vi "Do.vi"(8 "error in (no error)":errorcluster, 10 "Series Enqueuer":refnum<class "Message Enqueuer.lvclass">, 11 "Sample PID Light in":refnum<class "Sample PID Light.lvclass">) -> (0 "error out":errorcluster, 3 "Sample PID Light out":refnum<class "Sample PID Light.lvclass">)   [LabVIEW 2023, in "Sample PID Light.lvclass"]
uses:
  Sample PID Light.lvclass
  D:/git/HAL/HAL GOOP4/Task/Task Base/Task Base.lvclass
  <vilib>/ActorFramework/Message Enqueuer/Message Enqueuer.lvclass
  Task/Task Base/Task Base.lvclass/Task Base.ctl
  Series/ISeries Actor/ISeries Actor Messages/Point Data Updated Msg/Point Data Updated Msg.lvclass/Point Data Updated Msg.ctl
  <vilib>/ActorFramework/Message Enqueuer/Message Enqueuer.lvclass/Message Enqueuer.ctl
  <vilib>/ActorFramework/Message Enqueuer/Enqueue.vi
  Series/ISeries Actor/ISeries Actor Messages/Point Data Updated Msg/Point Data Updated Msg.lvclass
  C:/Program Files/National Instruments/LabVIEW 2023/vi.lib/ActorFramework/Message/Message.lvclass
  <vilib>/addons/control/pid/pid.llb/PID (DBL).vi
  <vilib>/Utility/LVClass/Get LV Class Name.vi
  <resource>/AFDebug/Generate Trace for Message.vi
  <vilib>/ActorFramework/Message Priority Queue/Priority Enqueue.vi
  Task/Task Base/Task Base.lvclass
  <vilib>/addons/control/pid/NI_PID_pid.lvlib
  Measure and Stimulus Subsystems/Measure and Stimulus Subsystems.lvclass
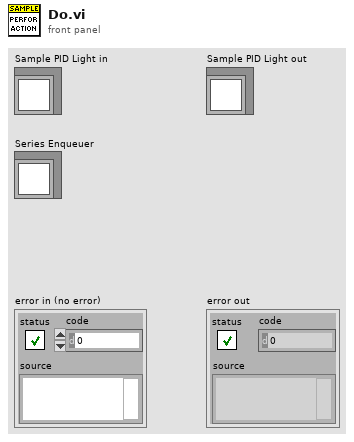
[diagram p1: front panel]
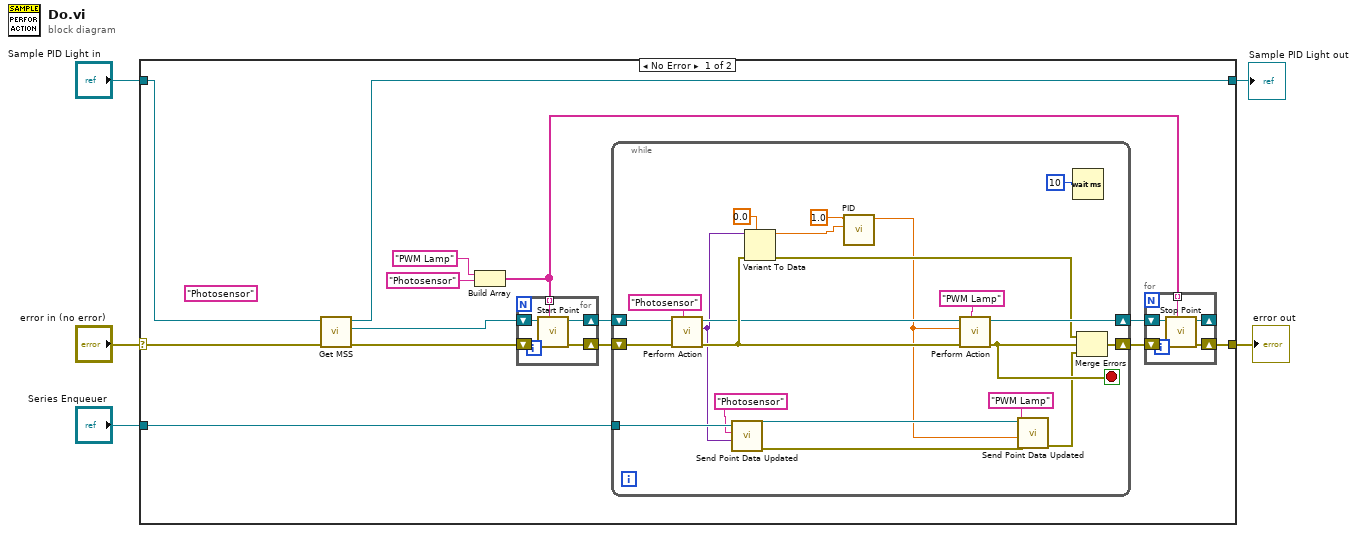
[diagram p0: block diagram]
diagram:
  n1 = case shown="No Error" "error in (no error)" {
    selector: "error in (no error)" -> [w16 w53]
    tunnel: [w12 w53] -> w3
    tunnel: [w7 w52] -> w2
    tunnel: "Sample PID Light in" -> [w8 w52]
    tunnel: "Series Enqueuer" -> [w6 _]
    frame No Error {
      (unwired) "Photosensor" ("Name")
      n2 = call "Get MSS.vi"("error in (no error)"=w16, "Task Base in"=w8) -> ("error out"=w15:errorcluster, "MSS"=w14:refnum<class "Measure and Stimulus Subsystems.lvclass">, "Task Base out"=w7:refnum<class "Sample PID Light.lvclass">)  [unwired: 7 in]
      n3 = Build Array("PWM Lamp" ("Target Ident"), "Photosensor" ("Target Identifier")) -> (w9:string[])
      n4 = for {
        shift-right: [w24] -> w19
        shift-left: w15 -> [w22]
        shift-right: [w23] -> w18
        shift-left: w14 -> [w21]
        tunnel: w9 -> [w20] mode=indexing
        n5 = call "Start Point.vi"("Position Ident"=w20, "error in"=w22, "MSS in"=w21) -> ("error out"=w24:errorcluster, "MSS out"=w23:refnum<class "Measure and Stimulus Subsystems.lvclass">)  [unwired: 7 in]
      }
      n6 = while {
        shift-right: [w38] -> w17
        shift-left: w19 -> [w42]
        shift-right: [w44] -> w13
        shift-left: w18 -> [w41]
        tunnel: w6 -> [w29]
        stop <- w36 stop-if-true
        n7 = call "Perform Action.vi"("Point Ident"="Photosensor" ("Target Identifier"), "error in"=w42, "MSS in"=w41) -> ("error out"=w34:errorcluster, "Output"=w27:variant, "MSS out"=w33:refnum<class "Measure and Stimulus Subsystems.lvclass">)  [unwired: 6 in]
        n8 = call "Send Point Data Updated.vi"("Data"=w27, "Point Ident"="Photosensor" ("Target Identifier"), "Message Enqueuer"=w29) -> ("error out"=w31:errorcluster, "Message Enqueuer out"=w32:refnum<class "Message Enqueuer.lvclass">)  [unwired: 7 in]
        n9 = Variant To Data(error in=w34, type=0.0, Variant=w27) -> (data=w39:dbl, error out=w37:errorcluster)
        n10 = call-poly <vilib>:"PID.vi"("process variable"=w39, "setpoint"=1.0) -> ("output"=w28:dbl)  [unwired: 8 in, 1 out]
        n11 = call "Perform Action.vi"("Point Ident"="PWM Lamp" ("Target Ident"), "error in"=w34, "Input"=w28, "MSS in"=w33) -> ("error out"=w36:errorcluster, "MSS out"=w44:refnum<class "Measure and Stimulus Subsystems.lvclass">)  [unwired: 5 in, 1 out]
        n12 = call "Send Point Data Updated.vi"("error in (no error)"=w31, "Data"=w28, "Point Ident"="PWM Lamp" ("Target Ident"), "Message Enqueuer"=w32) -> ("error out"=w25:errorcluster)  [unwired: 6 in, 1 out]
        n13 = Wait (ms)(milliseconds to wait=u32 10) -> ()  [unwired: 1 out]
        n14 = Merge Errors(w37, w36, w25) -> (w38:errorcluster)
      }
      n15 = for {
        shift-right: [w49] -> w12
        shift-left: w17 -> [w51]
        tunnel: w9 -> [w47] mode=indexing
        shift-right: [w48] -> _
        shift-left: w13 -> [w50]
        n16 = call "Stop Point.vi"("Point Ident"=w47, "error in"=w51, "MSS in"=w50) -> ("error out"=w49:errorcluster, "MSS out"=w48:refnum<class "Measure and Stimulus Subsystems.lvclass">)  [unwired: 7 in]
      }
    }
    frame Error {
    }
  }
  "error out" <- w3
  "Sample PID Light out" <- w2
